vi "Update Button Press on UI.vi"(0 "GEA2 Reference In":refnum<k24>, 5 "Test Results in":T1, 11 "error in (no error)":errorcluster) -> (4 "GEA2 Reference Out":refnum<k24>, 6 "Test Results out":T1, 15 "error out":errorcluster)   [LabVIEW 2016]
doc: "This VI reads the Button Press ERD and Button History ERD in order to update the UI."
uses:
  controls/Test Results.ctl
  C:/Automation/DLLs/PC Dot Net/GeaCommunication.dll
  Common/LabVIEW GEA2 Toolkit/LabVIEW_GEA2_Toolkit.lvlibp/type defs/ERD Read Data In.ctl
  Common/LabVIEW GEA2 Toolkit/LabVIEW_GEA2_Toolkit.lvlibp/type defs/Data Type.ctl
  Common/LabVIEW GEA2 Toolkit/LabVIEW_GEA2_Toolkit.lvlibp/type defs/Source_Destination.ctl
  Common/LabVIEW GEA2 Toolkit/LabVIEW_GEA2_Toolkit.lvlibp
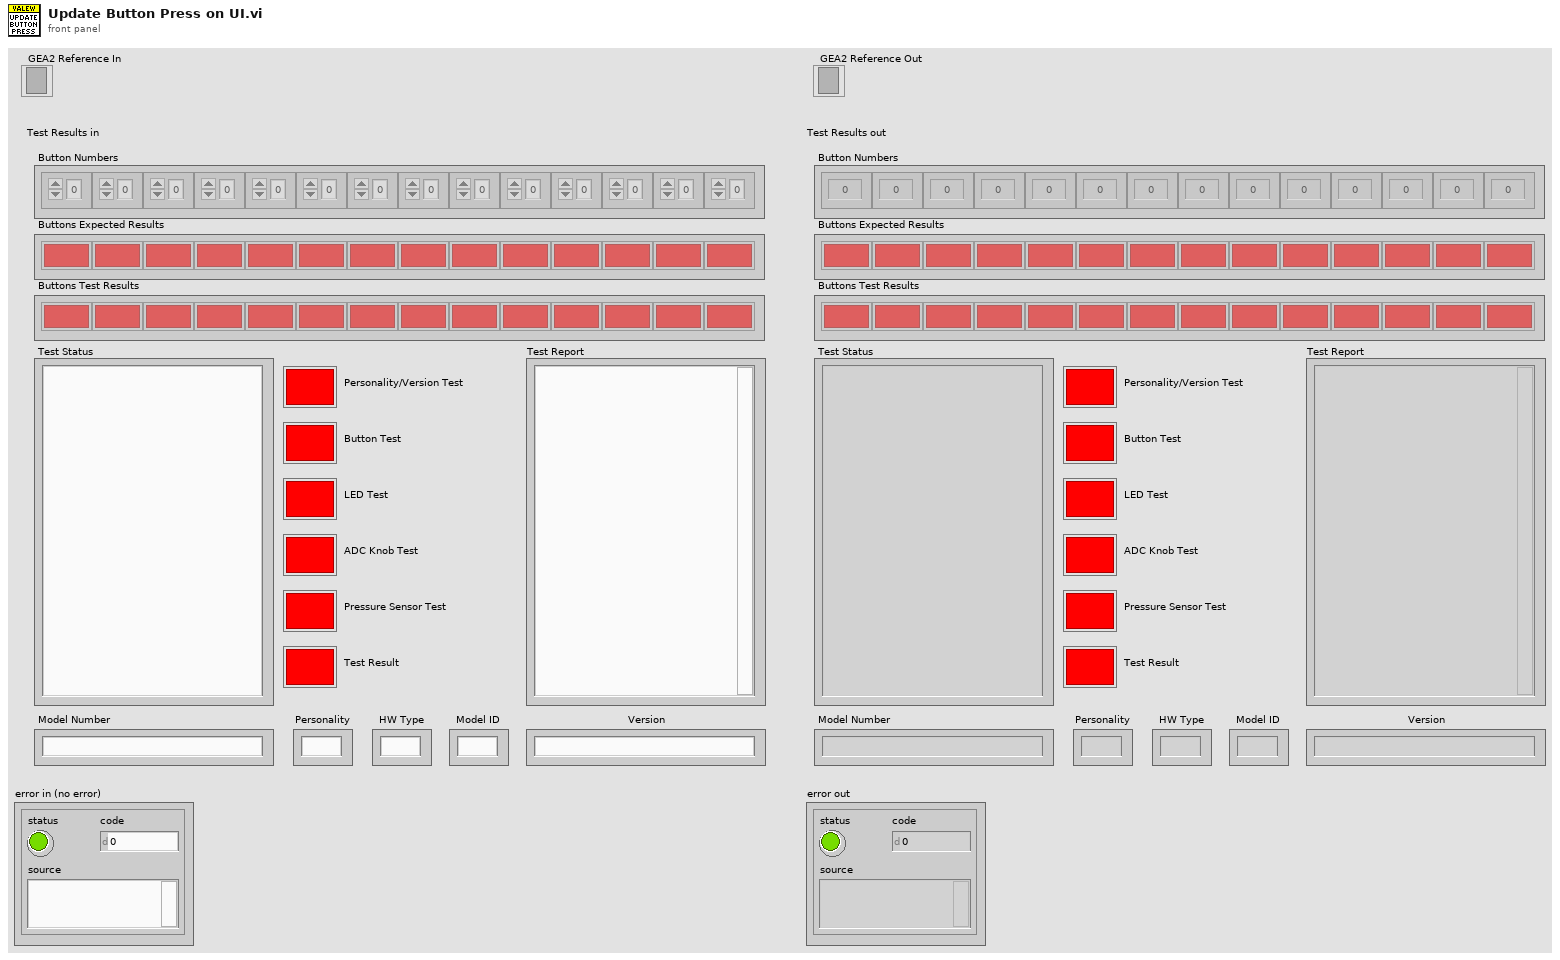
[diagram p1: front panel]
types:
  T1 = typedef "Test Results.ctl" = cluster{"Test Status":string, "Personality/Version Test ":bool, "Test Report":string, "Model Number":string, "Button Numbers":i32[], "Buttons Test Results":bool[], "Buttons Expected Results":bool[], "Model ID":string, "Personality":string, "HW Type":string, "Version":string, "Button Test":bool, "LED Test":bool, "ADC Knob Test":bool, "Pressure Sensor Test":bool, "Test Result":bool}
  T2 = typedef "LabVIEW_GEA2_Toolkit.lvlibp/Source_Destination.ctl" = cluster{"Source":u8, "Destination":u8}
  T3 = typedef "LabVIEW_GEA2_Toolkit.lvlibp/ERD Read Data In.ctl" = cluster{"ERD Number":u16, "Data Type":T4}
  T4 = typedef "LabVIEW_GEA2_Toolkit.lvlibp/Data Type.ctl" = enum16{"string", "boolean", "uint8_t", "uint16_t", "uint32_t", "uint64_t", "int8_t", "int16_t", "int32_t", "int64_t"}
  T5 = typedef "LabVIEW_GEA2_Toolkit.lvlibp/ERD Read Data Out.ctl" = cluster{"ERD Number":u16, "Data":string}
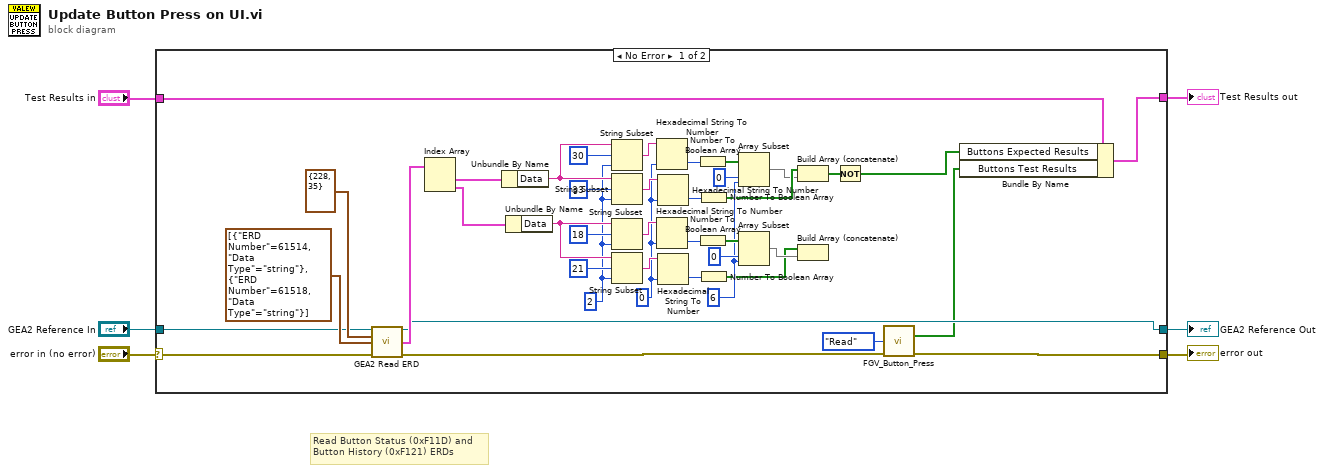
[diagram p0: block diagram]
diagram:
  # "Read Button Status (0xF11D) and \nButton History (0xF121) ERDs"
  n1 = case shown="No Error" "error in (no error)" {
    selector: "error in (no error)" -> [w37 w49]
    tunnel: [w46 w48] -> w6
    tunnel: "Test Results in" -> [w45 w48]
    tunnel: [w9 w49] -> w4
    tunnel: [w39 w50] -> w3
    tunnel: "GEA2 Reference In" -> [w38 w50]
    frame No Error {
      w16 = 6 ("length")
      w17 = u8 0
      w18 = 2 ("length (rest)")
      n2 = call "GEA2 Read ERD.vi"("GEA2 Reference In"=w38, "GEA Inputs"=T2 {"Source"=228, "Destination"=35}, "Read ERD List"=T3[] [{"ERD Number"=61514, "Data Type"=enum."string"}, {"ERD Number"=61518, "Data Type"=enum."string"}], "Error In"=w37) -> ("GEA2 Reference Out"=w39:refnum<k24>, "ERD Data Out"=w42:T5[], "Error Out"=w10:errorcluster)  [unwired: 8 in, 1 out]
      n3 = Index Array(array=w42) -> (element #1=w43:T5, element #2=w44:T5)  [unwired: 2 in]
      n4 = Unbundle By Name(w43) -> ("Data"=w34:string)
      n5 = Unbundle By Name(w44) -> ("Data"=w19:string)
      n6 = String Subset(string=w34, offset (0)=30, length (rest)=w18) -> (substring=w30:string)
      n7 = String Subset(string=w34, offset (0)=33, length (rest)=w18) -> (substring=w31:string)
      n8 = String Subset(string=w19, offset (0)=18, length (rest)=w18) -> (substring=w25:string)
      n9 = String Subset(string=w19, offset (0)=21, length (rest)=w18) -> (substring=w24:string)
      n10 = Hexadecimal String To Number(string=w30, default (0uL)=w17) -> (number=w33:u8)  [unwired: 1 in, 1 out]
      n11 = Hexadecimal String To Number(string=w25, default (0uL)=w17) -> (number=w22:u8)  [unwired: 1 in, 1 out]
      n12 = Hexadecimal String To Number(string=w31, default (0uL)=w17) -> (number=w32:u8)  [unwired: 1 in, 1 out]
      n13 = Hexadecimal String To Number(string=w24, default (0uL)=w17) -> (number=w23:u8)  [unwired: 1 in, 1 out]
      n14 = Number To Boolean Array(number=w33) -> (Boolean array=w29:bool[])
      n15 = Number To Boolean Array(number=w22) -> (Boolean array=w26:bool[])
      n16 = Number To Boolean Array(number=w32) -> (Boolean array=w14:bool[])
      n17 = Number To Boolean Array(number=w23) -> (Boolean array=w11:bool[])
      n18 = Array Subset(array=w29, index=0, length=w16) -> (w13:bool[])
      n19 = Array Subset(array=w26, index=0, length=w16) -> (w12:bool[])
      n20 = Build Array (concatenate)(w14, w13) -> (w15:bool[])
      n21 = Build Array (concatenate)(w11, w12) -> ()  [unwired: 1 out]
      n22 = Not(x=w15) -> (.not. x?=w47:bool[])
      n23 = call "FGV_Button_Press.vi"("Action"=enum16{"Read", "Write Stop", "Write Result"}."Read", "Error In"=w10) -> ("Boolean Array Out"=w7:bool[], "Error Out"=w9:errorcluster)  [unwired: 11 in, 1 out]
      n24 = Bundle By Name(cluster=w45, "Buttons Expected Results"=w47, "Buttons Test Results"=w7) -> (w46:T1)
    }
    frame Error {
    }
  }
  "Test Results out" <- w6
  "error out" <- w4
  "GEA2 Reference Out" <- w3
